vi "Joy_Adjust.vi"(7 "Rotation Special Adjust?":bool, 9 "Rotation":dbl, 10 "Y":dbl, 11 "X":dbl) -> (1 "Rotation'":dbl, 2 "Y'":dbl, 3 "X'":dbl)   [LabVIEW 2017]
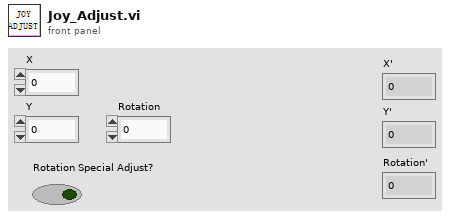
[diagram p1: front panel]
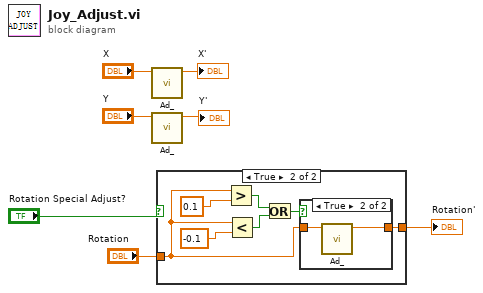
[diagram p0: block diagram]
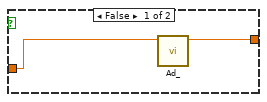
[diagram p2: hidden frame]
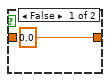
[diagram p3: hidden frame]
diagram:
  n1 = call "Ad_.vi"("X"="X") -> ("X'"=→"X'":dbl)  [unwired: 10 in]
  n2 = call "Ad_.vi"("X"="Y") -> ("X'"=→"Y'":dbl)  [unwired: 10 in]
  n3 = case shown="True" "Rotation Special Adjust?" {
    tunnel: "Rotation" -> [w9 w11]
    tunnel: [w8 w10] -> w1
    frame False {
      n4 = call "Ad_.vi"("X"=w9) -> ("X'"=w8:dbl)  [unwired: 10 in]
    }
    frame True {
      n5 = Greater?(x=w11, y=0.1) -> (0:w14:bool)
      n6 = Less?(x=w11, y=-0.1) -> (x < y?=w16:bool)
      n7 = Or(x=w14, y=w16) -> (x .or. y?=w15:bool)
      n8 = case shown="True" w15 {
        tunnel: [0.0 w18] -> w10
        tunnel: w11 -> [_ w19]
        frame False {
        }
        frame True {
          n9 = call "Ad_.vi"("X"=w19) -> ("X'"=w18:dbl)  [unwired: 10 in]
        }
      }
    }
  }
  "Rotation'" <- w1
